vi "Get Barometer Data V.vi"(8 "error in (no error)":errorcluster, 11 "barCalData":T1) -> (0 "error out":errorcluster, 2 "function return":i16, 3 "barCalData out":T1)   [LabVIEW 2009, in "VantagePro.lvlib"]
doc: "DllAccess short int _stdcall GetBarometerData_V ( BarCalData *barCalData);"
uses:
  VantagePro.lvlib
  <userlib>/VantagePro/VantagePro.dll
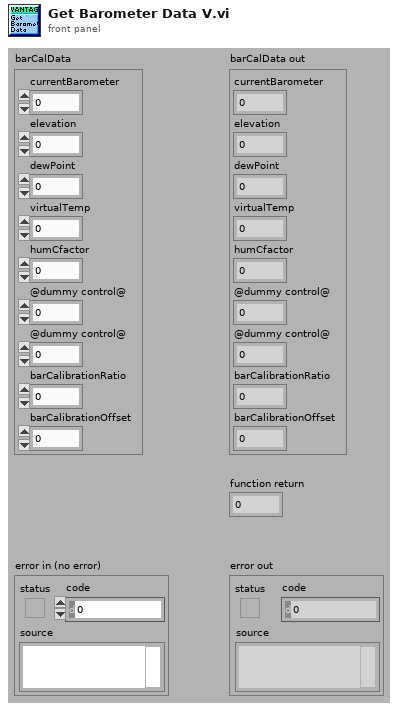
[diagram p1: front panel]
types:
  T1 = cluster{"currentBarometer":sgl, "elevation":sgl, "dewPoint":sgl, "virtualTemp":sgl, "humCfactor":i16, "@dummy control@":i8, "@dummy control@":i8, "barCalibrationRatio":sgl, "barCalibrationOffset":sgl}
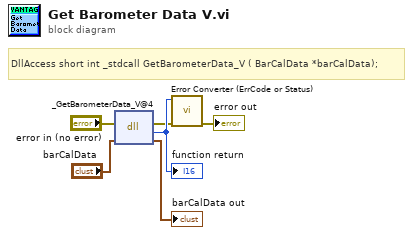
[diagram p0: block diagram]
diagram:
  # "DllAccess short int _stdcall GetBarometerData_V ( BarCalData *barCalData);"
  n1 = dll-call lib="C:/Program Files/National Instruments/LabVIEW 2010/user.lib/VantagePro/VantagePro.*" fn="_GetBarometerData_V@4"(error in="error in (no error)", "barCalData"="barCalData") -> (error out=w2:errorcluster, w6:i16, "barCalData"=→"barCalData out":T1)  [unwired: 2 in, 1 out]
  "function return" <- w6
  n2 = call "Error Converter (ErrCode or Status).vi"("error in (no error)"=w2, "error code"=w6) -> ("error out"=→"error out":errorcluster)  [unwired: 9 in]
